vi "GuiderSetupGUI.vi"() -> ()   [LabVIEW 2018]
uses:
  GuiderSetup/GuiderSetup.lvclass
  C:/Users/devstaff/sparc4/s4gui/Versao ZeroMQ REQ-REP/SPARC4_GUI -20241104/S4GUI/S4GUI.lvclass
  S4GUI/S4GUI.lvclass/S4GUI.ctl
  Instrument/Instrument.lvclass/Instrument.ctl
  Device/Optics/Optics.lvclass/Optics.ctl
  Device/Optics/Opt_Continuous/Opt_Continuous.lvclass
  C:/Users/devstaff/sparc4/s4gui/Versao ZeroMQ REQ-REP/SPARC4_GUI -20241104/Device/Optics/Optics.lvclass
  Instrument/Instrument.lvclass
  AG/AG.lvclass
  Device/angles/angles.lvclass
  S4GUI/S4GUI.lvclass
  Device/Optics/Optics.lvclass
  StateMachine/State Machine.lvclass
panel:
  out "GUI version":string
  in  "Tab Focus":enum32{"FOCUS", "Config"}(tab)
  in  "Guider Focus Target":dbl caption="Target" min=0.0 max=24.9 step=0.1
  in  "GOTO GFOC":bool
  in  "STOP GFOC":bool
  in  "GFOC IN":bool
  in  "GFOC OUT":bool
  out "Pos GFOC":dbl caption="Position (mm)" format="%3_4g"
  out "GFOC status":bool
  in  "Guider Focus Incr":dbl caption="Increment" min=0.0 max=5.0 step=0.01 format="%#2_4g"
  in  "Set Focus by Mode":bool
  in  "Focus by Mode":T1={"Phot."=17.0, "Polarim"=7.0, "Efficiency"=0.0, "Instrumental"=0.0}
  out "AG connection":bool caption="AG"
  in  "Rotator":dbl caption="ROTATOR"
  out "loop max (ms)":u32
  out "loop time (ms)":u32
  in  "Guider Mirror Veloc":dbl=1.0 caption="Veloc. (1-30)" min=1.0 max=30.0 step=1.0
  out "GMIR status":bool
  out "ICS connection":bool caption="ICS"
  out "error out":errorcluster
  out "Pos GMIR":dbl caption="Position (deg)" format="%-3_4g"
  in  "RUN GMIR":bool
  in  "STOP GMIR":bool
  in  "GOTO GMIR":bool
  in  "Guider Mirror Target":dbl caption="Target"
  in  "stop":bool
  in  "GuiderSetup.lvclass":refnum<class "GuiderSetup.lvclass">
  # "GUIDER SETUP"
  # "MIRROR"
  # "deg"
  # "deg/s"
  # "FOCUS"
  # "mm"
  # "mm"
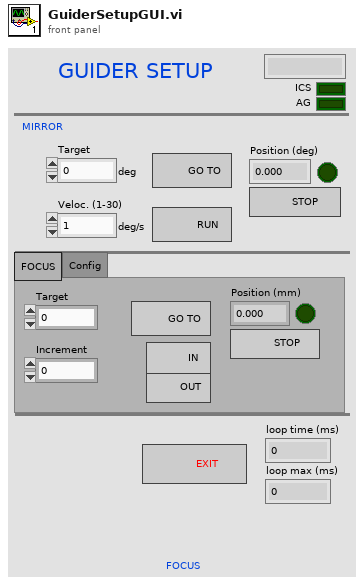
[diagram p1: front panel]
types:
  T1 = cluster{"Phot.":dbl, "Polarim":dbl, "Efficiency":dbl, "Instrumental":dbl}
  T2 = cluster{"Trigger Mode Status":string, "String output":string, "Instrument Status":cluster{"WPROT pos":dbl, "WPSEL pos":dbl, "GMIR pos":dbl, "GFOC pos":dbl, "CALW pos":dbl, "ASEL pos":dbl, "mode":bool, "String Status":string, "connection":bool, "operational":bool}, "Sync Box State":i32, "Trigger General Status":string, "Instrument States":cluster{"WPSEL State":i32, "WPROT State":i32, "CALW State":i32, "ASEL State":i32, "GMIR State":i32, "GFOC State":i32}, "Instrument Pos Names":cluster{"WPROT posname":string, "WPSEL posname":string, "CALW posname":string, "ASEL posname":string}, "ChannelA_Status":cluster{"Current exp":dbl, "Frames done":u32, "LastFileImage":string, "CamStatus":string, "Run state":u32, "connection":bool, "Cooler ON/OFF":i16, "Currently temperature":i16, "Temperature Status":string, "target  temp":i16, "conf runing":bool, "FT":bool, "UsedDisk":u16, "operational":bool}, "WPROT seq":u16, "ChannelB_Status":cluster{"Current exp":dbl, "Frames done":u32, "LastFileImage":string, "CamStatus":string, "Run state":u32, "connection":bool, "Cooler ON/OFF":i16, "Currently temperature":i16, "Temperature Status":string, "target  temp":i16, "conf runing":bool, "FT":bool, "UsedDisk":u16, "operational":bool}, "ChannelC_Status":cluster{"Current exp":dbl, "Frames done":u32, "LastFileImage":string, "CamStatus":string, "Run state":u32, "connection":bool, "Cooler ON/OFF":i16, "Currently temperature":i16, "Temperature Status":string, "target  temp":i16, "conf runing":bool, "FT":bool, "UsedDisk":u16, "operational":bool}, "ChannelD_Status":cluster{"Current exp":dbl, "Frames done":u32, "LastFileImage":string, "CamStatus":string, "Run state":u32, "connection":bool, "Cooler ON/OFF":i16, "Currently temperature":i16, "Temperature Status":string, "target  temp":i16, "conf runing":bool, "FT":bool, "UsedDisk":u16, "operational":bool}, "ChannelA_CCD":cluster{"ACQUISITION_MODE":u8, "TRIGGER_MODE":u8, "READ_MODE":u8, "PREAMP":u8, "READOUT_RATE":u8, "VERTICAL_SHIFT_SPEED":u8, "EM_MODE":u8, "EM_GAIN":u16, "SHUTTER_MODE":u8, "SHUTTER_TTL":u8, "SHUTTER_OPENNING_TIME":u16, "SHUTTER_CLOSING_TIME":u16, "VBIN":u16, "HBIN":u16, "INITIAL_LINE":u16, "INITIAL_COLUMN":u16, "FINAL_LINE":u16, "FINAL_COLUMN":u16, "FRAME_TRANSFER":bool, "VERTICAL_CLOCK_VOLTAGE":u8, "AD_CHANNEL":u32}, "ChannelB_CCD ":cluster{"ACQUISITION_MODE":u8, "TRIGGER_MODE":u8, "READ_MODE":u8, "PREAMP":u8, "READOUT_RATE":u8, "VERTICAL_SHIFT_SPEED":u8, "EM_MODE":u8, "EM_GAIN":u16, "SHUTTER_MODE":u8, "SHUTTER_TTL":u8, "SHUTTER_OPENNING_TIME":u16, "SHUTTER_CLOSING_TIME":u16, "VBIN":u16, "HBIN":u16, "INITIAL_LINE":u16, "INITIAL_COLUMN":u16, "FINAL_LINE":u16, "FINAL_COLUMN":u16, "FRAME_TRANSFER":bool, "VERTICAL_CLOCK_VOLTAGE":u8, "AD_CHANNEL":u32}, "ChannelC_CCD":cluster{"ACQUISITION_MODE":u8, "TRIGGER_MODE":u8, "READ_MODE":u8, "PREAMP":u8, "READOUT_RATE":u8, "VERTICAL_SHIFT_SPEED":u8, "EM_MODE":u8, "EM_GAIN":u16, "SHUTTER_MODE":u8, "SHUTTER_TTL":u8, "SHUTTER_OPENNING_TIME":u16, "SHUTTER_CLOSING_TIME":u16, "VBIN":u16, "HBIN":u16, "INITIAL_LINE":u16, "INITIAL_COLUMN":u16, "FINAL_LINE":u16, "FINAL_COLUMN":u16, "FRAME_TRANSFER":bool, "VERTICAL_CLOCK_VOLTAGE":u8, "AD_CHANNEL":u32}, "ChannelD_CCD":cluster{"ACQUISITION_MODE":u8, "TRIGGER_MODE":u8, "READ_MODE":u8, "PREAMP":u8, "READOUT_RATE":u8, "VERTICAL_SHIFT_SPEED":u8, "EM_MODE":u8, "EM_GAIN":u16, "SHUTTER_MODE":u8, "SHUTTER_TTL":u8, "SHUTTER_OPENNING_TIME":u16, "SHUTTER_CLOSING_TIME":u16, "VBIN":u16, "HBIN":u16, "INITIAL_LINE":u16, "INITIAL_COLUMN":u16, "FINAL_LINE":u16, "FINAL_COLUMN":u16, "FRAME_TRANSFER":bool, "VERTICAL_CLOCK_VOLTAGE":u8, "AD_CHANNEL":u32}, "CHA_Checked Params":cluster{"ACQUISITION_MODE":bool, "TRIGGER_MODE":bool, "READ_MODE":bool, "PREAMP":bool, "READOUT_RATE":bool, "VERTICAL_SHIFT_SPEED":bool, "EM_MODE":bool, "EM_GAIN":bool, "SHUTTER_MODE":bool, "SHUTTER_TTL":bool, "SHUTTER_OPENING_TIME":bool, "SHUTTER_CLOSING_TIME":bool, "VBIN":bool, "HBIN":bool, "INITIAL_LINE":bool, "INITIAL_COLUMN":bool, "FINAL_LINE":bool, "FINAL_COLUMN":bool, "FRAME_TRANSFER":bool, "VERTICAL_CLOCK_VOLTAGE":bool, "AD_CHANNEL":bool}, "CHB_Checked Params":cluster{"ACQUISITION_MODE":bool, "TRIGGER_MODE":bool, "READ_MODE":bool, "PREAMP":bool, "READOUT_RATE":bool, "VERTICAL_SHIFT_SPEED":bool, "EM_MODE":bool, "EM_GAIN":bool, "SHUTTER_MODE":bool, "SHUTTER_TTL":bool, "SHUTTER_OPENING_TIME":bool, "SHUTTER_CLOSING_TIME":bool, "VBIN":bool, "HBIN":bool, "INITIAL_LINE":bool, "INITIAL_COLUMN":bool, "FINAL_LINE":bool, "FINAL_COLUMN":bool, "FRAME_TRANSFER":bool, "VERTICAL_CLOCK_VOLTAGE":bool, "AD_CHANNEL":bool}, "CHC_Checked Params":cluster{"ACQUISITION_MODE":bool, "TRIGGER_MODE":bool, "READ_MODE":bool, "PREAMP":bool, "READOUT_RATE":bool, "VERTICAL_SHIFT_SPEED":bool, "EM_MODE":bool, "EM_GAIN":bool, "SHUTTER_MODE":bool, "SHUTTER_TTL":bool, "SHUTTER_OPENING_TIME":bool, "SHUTTER_CLOSING_TIME":bool, "VBIN":bool, "HBIN":bool, "INITIAL_LINE":bool, "INITIAL_COLUMN":bool, "FINAL_LINE":bool, "FINAL_COLUMN":bool, "FRAME_TRANSFER":bool, "VERTICAL_CLOCK_VOLTAGE":bool, "AD_CHANNEL":bool}, "CHD_Checked Params":cluster{"ACQUISITION_MODE":bool, "TRIGGER_MODE":bool, "READ_MODE":bool, "PREAMP":bool, "READOUT_RATE":bool, "VERTICAL_SHIFT_SPEED":bool, "EM_MODE":bool, "EM_GAIN":bool, "SHUTTER_MODE":bool, "SHUTTER_TTL":bool, "SHUTTER_OPENING_TIME":bool, "SHUTTER_CLOSING_TIME":bool, "VBIN":bool, "HBIN":bool, "INITIAL_LINE":bool, "INITIAL_COLUMN":bool, "FINAL_LINE":bool, "FINAL_COLUMN":bool, "FRAME_TRANSFER":bool, "VERTICAL_CLOCK_VOLTAGE":bool, "AD_CHANNEL":bool}, "Trigger_connection":bool, "TCSPD_connection":bool, "TCS extended":string, "TCS id":u32, "S4ICS id":u32, "focus pos":i32, "Focus_connection":bool, "WS_connection":bool, "weather status":cluster{"broker":string, "version":string, "date":string, "hour":string, "outHumidity":string, "inHumidity":string, "inTemp":string, "outTemp":string, "windSpeed":string, "windDirection":string, "pressure":string, "dewOut":string, "dewIn":string, "leaf":string, "rain":string, "windChill":string}, "GS STATUS cluster":cluster{"FocusPhot":dbl, "FocusPolar":dbl, "FocusEffic":dbl, "FocusInstrum":dbl, "ICS":bool, "AG":bool, "BROKER":string}, "TCSPD_operational":bool, "Focus_operational":bool}
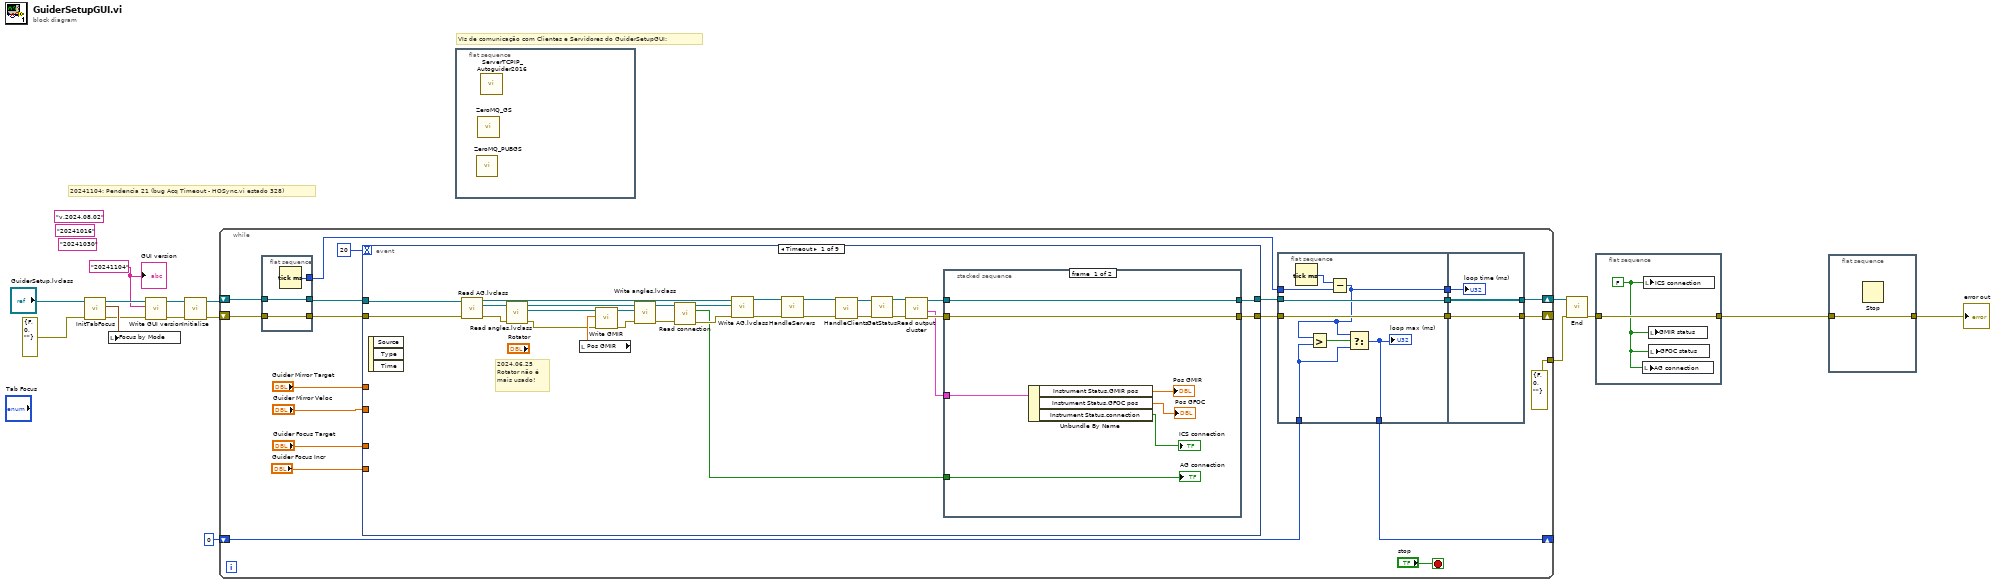
[diagram p0: block diagram]
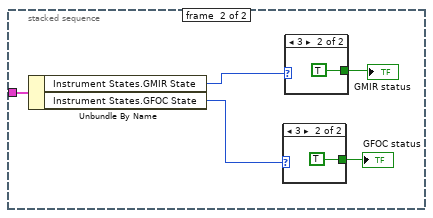
[diagram p2: hidden frame]
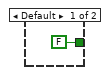
[diagram p3: hidden frame]
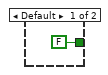
[diagram p4: hidden frame]
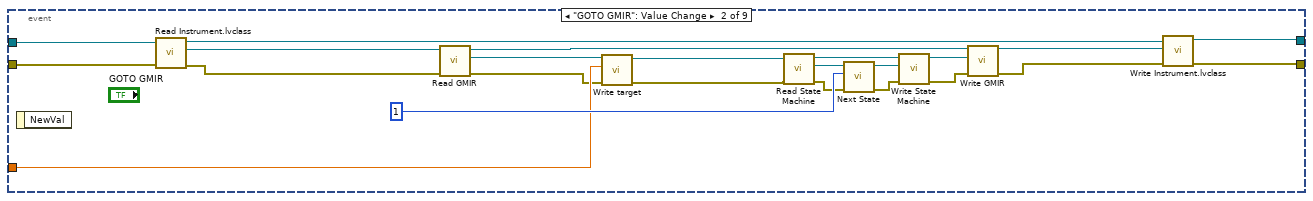
[diagram p5: hidden frame]
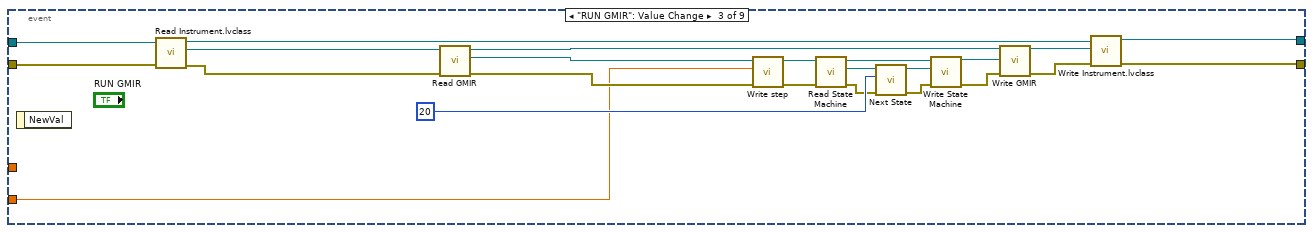
[diagram p6: hidden frame]
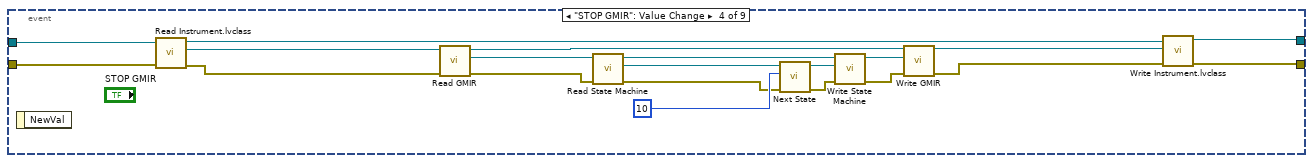
[diagram p7: hidden frame]
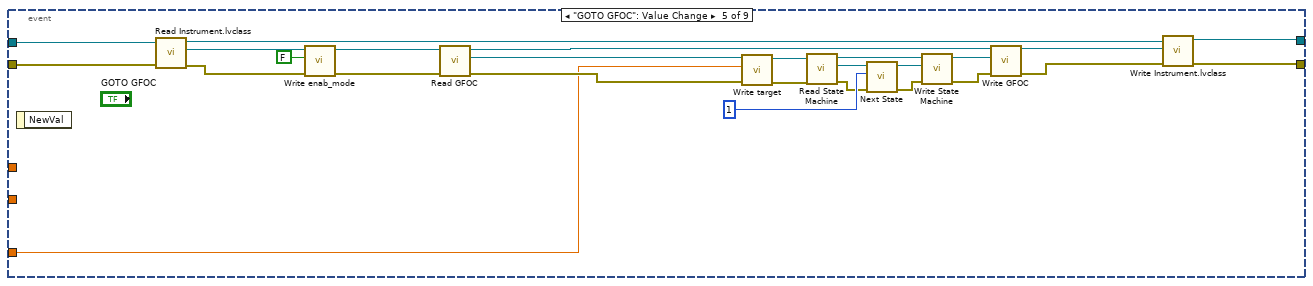
[diagram p8: hidden frame]
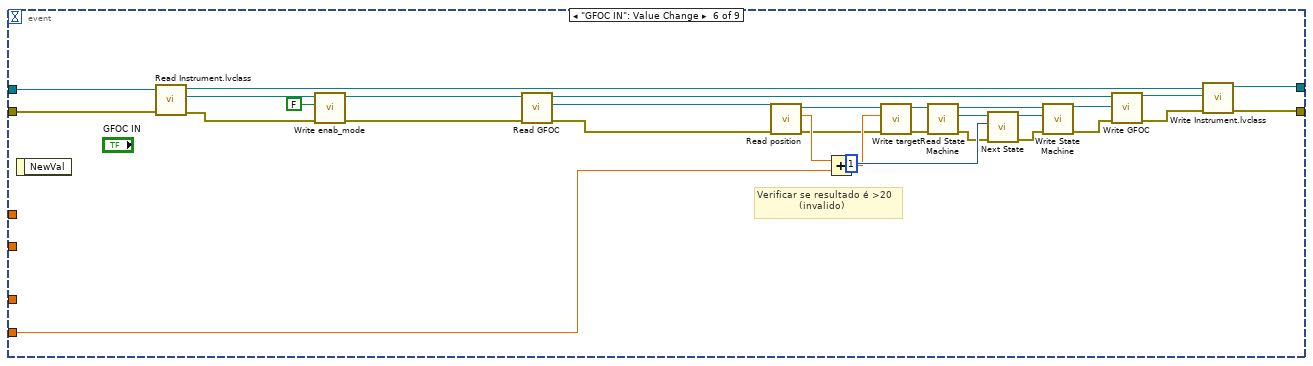
[diagram p9: hidden frame]
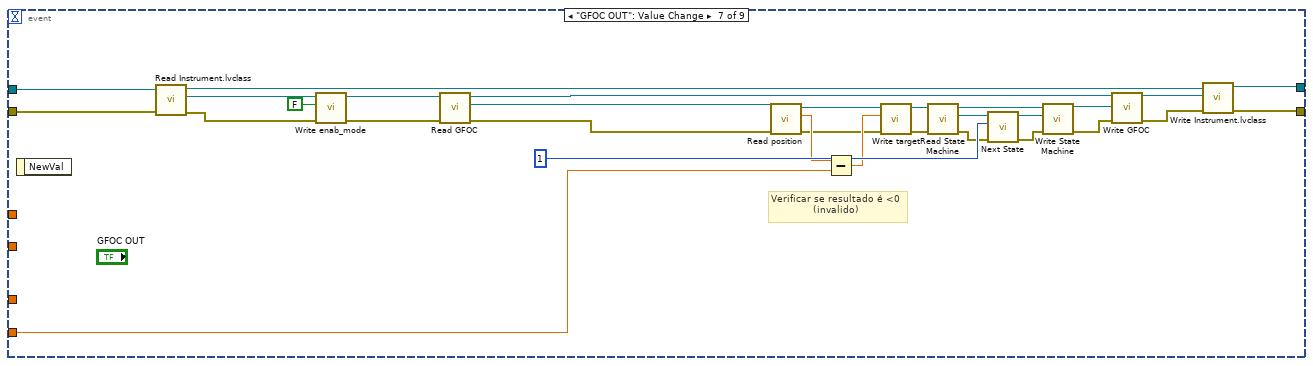
[diagram p10: hidden frame]
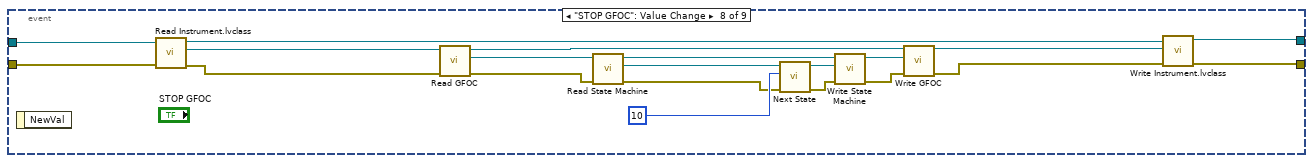
[diagram p11: hidden frame]
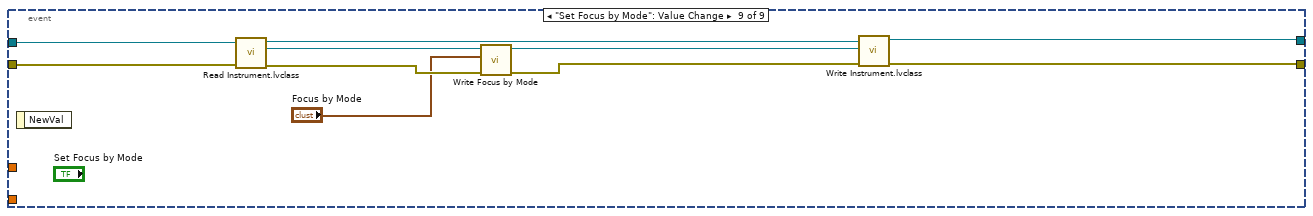
[diagram p12: hidden frame]
diagram:
  (unwired) "20241030" ("GUI version")
  (unwired) "20241016" ("GUI version")
  w1 = "20241104" ("GUI version")
  (unwired) "v.2024.08.02" ("GUI version")
  # "20241104: Pendencia 21 (bug Acq Timeout - HOSync.vi estado 328)"
  # "VIs de comunicação com Clientes e Servidores do GuiderSetupGUI:"
  n1 = call-dynamic "InitTabFocus.vi"("error in (no error)"=errorcluster {"status"=FALSE, "code"=0, "source"=""}, "GuiderSetup in"="GuiderSetup.lvclass") -> ("error out"=w5:errorcluster, "output cluster"=w8:T1, "GuiderSetup out"=w7:refnum<class "GuiderSetup.lvclass">)  [unwired: 7 in]
  n2 = local write "Focus by Mode"(w8) -> ()
  n3 = call-dynamic "Write GUI version.vi"("error in (no error)"=w5, "GUI version"=w1, "S4GUI in"=w7) -> ("error out"=w4:errorcluster, "S4GUI out"=w6:refnum<class "GuiderSetup.lvclass">)  [unwired: 7 in]
  n4 = call-dynamic "Initialize.vi"("error in (no error)"=w4, "S4ACS_GUI in"=w6) -> ("error out"=w15:errorcluster, "S4ACS_GUI out"=w16:refnum<class "GuiderSetup.lvclass">)  [unwired: 8 in]
  n5 = while {
    shift-right: [w24] -> w14
    shift-left: w16 -> [w31]
    shift-right: [w25] -> _
    shift-left: w15 -> [w30]
    shift-right: [w19] -> _
    shift-left: u32 0 -> [w18]
    tunnel: [errorcluster {"status"=FALSE, "code"=0, "source"=""} ("error in (no error)")] -> w11
    stop <- "stop" stop-if-true
    n6 = flat-sequence {
      tunnel: [w51] -> w20
      tunnel: w31 -> [w50]
      tunnel: w30 -> [w49]
      tunnel: [w50] -> w29
      tunnel: [w49] -> w28
      frame #0 {
        n7 = Tick Count (ms)() -> (millisecond timer value=w51:u32)
      }
    }
    n8 = event shown="[0] Timeout" {
      selector: _ -> [_ _ _ _ _ _ _ _ _]
      dyn-events: _ -> [_ _ _ _ _ _ _ _ _]
      timeout: 20 -> [_ _ _ _ _ _ _ _ _]
      tunnel: w29 -> [w80 w119 w142 w162 w188 w218 w248 w268 w278]
      tunnel: [w64 w117 w140 w160 w186 w216 w246 w266 w276] -> w27
      tunnel: w28 -> [w79 w113 w136 w156 w183 w213 w243 w262 w275]
      tunnel: [w61 w110 w133 w153 w181 w211 w241 w259 w274] -> w26
      tunnel: "Guider Mirror Veloc" -> [_ _ w120 _ _ _ _ _ _]
      tunnel: "Guider Mirror Target" -> [_ w99 _ _ _ _ _ _ _]
      tunnel: "Guider Focus Target" -> [_ _ _ _ w168 _ _ _ _]
      tunnel: "Guider Focus Incr" -> [_ _ _ _ _ w194 w224 _ _]
      event Timeout {
        # "2024.06.25\nRotator não é \nmais usado!"
        n9 = event-data() -> ()  [unwired: 1 in, 3 out]
        n10 = call-dynamic "Read AG.lvclass.vi"("error in (no error)"=w79, "GuiderSetup in"=w80) -> ("error out"=w74:errorcluster, "AG.lvclass"=w77:refnum<class "AG.lvclass">, "GuiderSetup out"=w78:refnum<class "GuiderSetup.lvclass">)  [unwired: 7 in]
        n11 = call-dynamic "Read angles.lvclass.vi"("error in (no error)"=w74, "AG in"=w77) -> ("error out"=w62:errorcluster, "angles.lvclass"=w63:refnum<class "angles.lvclass">, "AG out"=w76:refnum<class "AG.lvclass">)  [unwired: 7 in]
        n12 = local read "Pos GMIR"() -> (w72:dbl)
        n13 = call-dynamic "Write GMIR.vi"("error in (no error)"=w62, "GMIR"=w72, "angles in"=w63) -> ("error out"=w73:errorcluster, "angles out"=w75:refnum<class "angles.lvclass">)  [unwired: 7 in]
        n14 = call-dynamic "Write angles.lvclass.vi"("error in (no error)"=w73, "angles.lvclass"=w75, "AG in"=w76) -> ("error out"=w67:errorcluster, "AG out"=w69:refnum<class "AG.lvclass">)  [unwired: 7 in]
        n15 = call-dynamic "Read connection.vi"("error in (no error)"=w67, "Client in"=w69) -> ("error out"=w66:errorcluster, "connection"=w65:bool, "Client out"=w68:refnum<class "AG.lvclass">)  [unwired: 7 in]
        n16 = call-dynamic "Write AG.lvclass.vi"("error in (no error)"=w66, "AG.lvclass"=w68, "GuiderSetup in"=w78) -> ("error out"=w71:errorcluster, "GuiderSetup out"=w70:refnum<class "GuiderSetup.lvclass">)  [unwired: 7 in]
        n17 = call-dynamic "HandleServers.vi"("error in (no error)"=w71, "S4ACS_GUI in"=w70) -> ("error out"=w58:errorcluster, "S4ACS_GUI out"=w60:refnum<class "GuiderSetup.lvclass">)  [unwired: 8 in]
        n18 = call-dynamic "HandleClients.vi"("error in (no error)"=w58, "GuiderSetup in"=w60) -> ("error out"=w57:errorcluster, "GuiderSetup out"=w59:refnum<class "GuiderSetup.lvclass">)  [unwired: 8 in]
        n19 = call-dynamic "GetStatus.vi"("error in (no error)"=w57, "GS in"=w59) -> ("error out"=w54:errorcluster, "GS out"=w56:refnum<class "GuiderSetup.lvclass">)  [unwired: 8 in]
        n20 = call-dynamic "Read output cluster.vi"("error in (no error)"=w54, "S4GUI in"=w56) -> ("error out"=w53:errorcluster, "output cluster"=w52:T2, "S4GUI out"=w55:refnum<class "GuiderSetup.lvclass">)  [unwired: 7 in]
        n21 = stacked-sequence {
          tunnel: w65 -> [w84 _]
          tunnel: w55 -> [w83 _]
          tunnel: w53 -> [w82 _]
          tunnel: [w83 _] -> w64
          tunnel: [w82 _] -> w61
          tunnel: w52 -> [w81 w88]
          frame #0 {
            n22 = Unbundle By Name(w81) -> ("Instrument Status.GMIR pos"=→"Pos GMIR":dbl, "Instrument Status.GFOC pos"=→"Pos GFOC":dbl, "Instrument Status.connection"=→"ICS connection":bool)
            "AG connection" <- w84
          }
          frame #1 {
            n23 = Unbundle By Name(w88) -> ("Instrument States.GMIR State"=w92:i32, "Instrument States.GFOC State"=w90:i32)
            n24 = case shown="3" w90 {
              tunnel: [FALSE TRUE] -> w89
              frame Default {
              }
              frame 3 {
              }
            }
            "GFOC status" <- w89
            n25 = case shown="3" w92 {
              tunnel: [FALSE TRUE] -> w91
              frame Default {
              }
              frame 3 {
              }
            }
            "GMIR status" <- w91
          }
        }
      }
      event "GOTO GMIR": Value Change {
        n26 = event-data() -> ()  [unwired: 1 in, 1 out]
        n27 = call "Read Instrument.lvclass.vi"("error in (no error)"=w113, "S4ACS_GUI in"=w119) -> ("error out"=w112:errorcluster, "Instrument.lvclass"=w116:refnum<class "Instrument.lvclass">, "S4ACS_GUI out"=w118:refnum<class "GuiderSetup.lvclass">)  [unwired: 7 in]
        n28 = call "Read GMIR.vi"("error in (no error)"=w112, "Instrument in"=w116) -> ("error out"=w98:errorcluster, "Opt_Continuous.lvclass"=w101:refnum<class "Opt_Continuous.lvclass">, "Instrument out"=w115:refnum<class "Instrument.lvclass">)  [unwired: 7 in]
        n29 = call "Write target.vi"("error in (no error)"=w98, "target"=w99, "Optics in"=w101) -> ("error out"=w97:errorcluster, "Optics out"=w100:refnum<class "Opt_Continuous.lvclass">)  [unwired: 7 in]
        n30 = call-dynamic "Read State Machine.vi"("error in (no error)"=w97, "Device in"=w100) -> ("error out"=w104:errorcluster, "State Machine.lvclass"=w107:refnum<class "State Machine.lvclass">, "Device out"=w109:refnum<class "Opt_Continuous.lvclass">)  [unwired: 7 in]
        n31 = call "Next State.vi"("error in (no error)"=w104, "New_State"=1, "State Machine in"=w107) -> ("error out"=w103:errorcluster, "State Machine out"=w106:refnum<class "State Machine.lvclass">)  [unwired: 7 in]
        n32 = call-dynamic "Write State Machine.vi"("error in (no error)"=w103, "State Machine.lvclass"=w106, "Device in"=w109) -> ("error out"=w102:errorcluster, "Device out"=w108:refnum<class "Opt_Continuous.lvclass">)  [unwired: 7 in]
        n33 = call "Write GMIR.vi"("error in (no error)"=w102, "Opt_Continuous.lvclass"=w108, "Instrument in"=w115) -> ("error out"=w111:errorcluster, "Instrument out"=w114:refnum<class "Instrument.lvclass">)  [unwired: 7 in]
        n34 = call "Write Instrument.lvclass.vi"("error in (no error)"=w111, "Instrument.lvclass"=w114, "S4ACS_GUI in"=w118) -> ("error out"=w110:errorcluster, "S4ACS_GUI out"=w117:refnum<class "GuiderSetup.lvclass">)  [unwired: 7 in]
      }
      event "RUN GMIR": Value Change {
        n35 = event-data() -> ()  [unwired: 1 in, 1 out]
        n36 = call "Read Instrument.lvclass.vi"("error in (no error)"=w136, "S4ACS_GUI in"=w142) -> ("error out"=w135:errorcluster, "Instrument.lvclass"=w139:refnum<class "Instrument.lvclass">, "S4ACS_GUI out"=w141:refnum<class "GuiderSetup.lvclass">)  [unwired: 7 in]
        n37 = call "Read GMIR.vi"("error in (no error)"=w135, "Instrument in"=w139) -> ("error out"=w123:errorcluster, "Opt_Continuous.lvclass"=w124:refnum<class "Opt_Continuous.lvclass">, "Instrument out"=w138:refnum<class "Instrument.lvclass">)  [unwired: 7 in]
        n38 = call-dynamic "Write step.vi"("error in (no error)"=w123, "step"=w120, "Optics in"=w124) -> ("error out"=w122:errorcluster, "Optics out"=w121:refnum<class "Opt_Continuous.lvclass">)  [unwired: 7 in]
        n39 = call-dynamic "Read State Machine.vi"("error in (no error)"=w122, "Device in"=w121) -> ("error out"=w127:errorcluster, "State Machine.lvclass"=w130:refnum<class "State Machine.lvclass">, "Device out"=w132:refnum<class "Opt_Continuous.lvclass">)  [unwired: 7 in]
        n40 = call "Next State.vi"("error in (no error)"=w127, "New_State"=20, "State Machine in"=w130) -> ("error out"=w126:errorcluster, "State Machine out"=w129:refnum<class "State Machine.lvclass">)  [unwired: 7 in]
        n41 = call-dynamic "Write State Machine.vi"("error in (no error)"=w126, "State Machine.lvclass"=w129, "Device in"=w132) -> ("error out"=w125:errorcluster, "Device out"=w131:refnum<class "Opt_Continuous.lvclass">)  [unwired: 7 in]
        n42 = call "Write GMIR.vi"("error in (no error)"=w125, "Opt_Continuous.lvclass"=w131, "Instrument in"=w138) -> ("error out"=w134:errorcluster, "Instrument out"=w137:refnum<class "Instrument.lvclass">)  [unwired: 7 in]
        n43 = call "Write Instrument.lvclass.vi"("error in (no error)"=w134, "Instrument.lvclass"=w137, "S4ACS_GUI in"=w141) -> ("error out"=w133:errorcluster, "S4ACS_GUI out"=w140:refnum<class "GuiderSetup.lvclass">)  [unwired: 7 in]
      }
      event "STOP GMIR": Value Change {
        n44 = event-data() -> ()  [unwired: 1 in, 1 out]
        n45 = call "Read Instrument.lvclass.vi"("error in (no error)"=w156, "S4ACS_GUI in"=w162) -> ("error out"=w155:errorcluster, "Instrument.lvclass"=w159:refnum<class "Instrument.lvclass">, "S4ACS_GUI out"=w161:refnum<class "GuiderSetup.lvclass">)  [unwired: 7 in]
        n46 = call "Read GMIR.vi"("error in (no error)"=w155, "Instrument in"=w159) -> ("error out"=w146:errorcluster, "Opt_Continuous.lvclass"=w152:refnum<class "Opt_Continuous.lvclass">, "Instrument out"=w158:refnum<class "Instrument.lvclass">)  [unwired: 7 in]
        n47 = call-dynamic "Read State Machine.vi"("error in (no error)"=w146, "Device in"=w152) -> ("error out"=w145:errorcluster, "State Machine.lvclass"=w149:refnum<class "State Machine.lvclass">, "Device out"=w151:refnum<class "Opt_Continuous.lvclass">)  [unwired: 7 in]
        n48 = call "Next State.vi"("error in (no error)"=w145, "New_State"=10, "State Machine in"=w149) -> ("error out"=w144:errorcluster, "State Machine out"=w148:refnum<class "State Machine.lvclass">)  [unwired: 7 in]
        n49 = call-dynamic "Write State Machine.vi"("error in (no error)"=w144, "State Machine.lvclass"=w148, "Device in"=w151) -> ("error out"=w143:errorcluster, "Device out"=w150:refnum<class "Opt_Continuous.lvclass">)  [unwired: 7 in]
        n50 = call "Write GMIR.vi"("error in (no error)"=w143, "Opt_Continuous.lvclass"=w150, "Instrument in"=w158) -> ("error out"=w154:errorcluster, "Instrument out"=w157:refnum<class "Instrument.lvclass">)  [unwired: 7 in]
        n51 = call "Write Instrument.lvclass.vi"("error in (no error)"=w154, "Instrument.lvclass"=w157, "S4ACS_GUI in"=w161) -> ("error out"=w153:errorcluster, "S4ACS_GUI out"=w160:refnum<class "GuiderSetup.lvclass">)  [unwired: 7 in]
      }
      event "GOTO GFOC": Value Change {
        n52 = event-data() -> ()  [unwired: 1 in, 1 out]
        n53 = call "Read Instrument.lvclass.vi"("error in (no error)"=w183, "S4ACS_GUI in"=w188) -> ("error out"=w166:errorcluster, "Instrument.lvclass"=w167:refnum<class "Instrument.lvclass">, "S4ACS_GUI out"=w187:refnum<class "GuiderSetup.lvclass">)  [unwired: 7 in]
        n54 = call-dynamic "Write enab_mode.vi"("error in (no error)"=w166, "enab_mode"=FALSE, "Instrument in"=w167) -> ("error out"=w163:errorcluster, "Instrument out"=w164:refnum<class "Instrument.lvclass">)  [unwired: 7 in]
        n55 = call "Read GFOC.vi"("error in (no error)"=w163, "Instrument in"=w164) -> ("error out"=w170:errorcluster, "Opt_Continuous.lvclass"=w172:refnum<class "Opt_Continuous.lvclass">, "Instrument out"=w185:refnum<class "Instrument.lvclass">)  [unwired: 7 in]
        n56 = call "Write target.vi"("error in (no error)"=w170, "target"=w168, "Optics in"=w172) -> ("error out"=w169:errorcluster, "Optics out"=w171:refnum<class "Opt_Continuous.lvclass">)  [unwired: 7 in]
        n57 = call-dynamic "Read State Machine.vi"("error in (no error)"=w169, "Device in"=w171) -> ("error out"=w175:errorcluster, "State Machine.lvclass"=w178:refnum<class "State Machine.lvclass">, "Device out"=w180:refnum<class "Opt_Continuous.lvclass">)  [unwired: 7 in]
        n58 = call "Next State.vi"("error in (no error)"=w175, "New_State"=1, "State Machine in"=w178) -> ("error out"=w174:errorcluster, "State Machine out"=w177:refnum<class "State Machine.lvclass">)  [unwired: 7 in]
        n59 = call-dynamic "Write State Machine.vi"("error in (no error)"=w174, "State Machine.lvclass"=w177, "Device in"=w180) -> ("error out"=w173:errorcluster, "Device out"=w179:refnum<class "Opt_Continuous.lvclass">)  [unwired: 7 in]
        n60 = call "Write GFOC.vi"("error in (no error)"=w173, "Opt_Continuous.lvclass"=w179, "Instrument in"=w185) -> ("error out"=w182:errorcluster, "Instrument out"=w184:refnum<class "Instrument.lvclass">)  [unwired: 7 in]
        n61 = call "Write Instrument.lvclass.vi"("error in (no error)"=w182, "Instrument.lvclass"=w184, "S4ACS_GUI in"=w187) -> ("error out"=w181:errorcluster, "S4ACS_GUI out"=w186:refnum<class "GuiderSetup.lvclass">)  [unwired: 7 in]
      }
      event "GFOC IN": Value Change {
        # "Verificar se resultado é >20 \n              (invalido)"
        n62 = event-data() -> ()  [unwired: 1 in, 1 out]
        n63 = call "Read Instrument.lvclass.vi"("error in (no error)"=w213, "S4ACS_GUI in"=w218) -> ("error out"=w191:errorcluster, "Instrument.lvclass"=w192:refnum<class "Instrument.lvclass">, "S4ACS_GUI out"=w217:refnum<class "GuiderSetup.lvclass">)  [unwired: 7 in]
        n64 = call-dynamic "Write enab_mode.vi"("error in (no error)"=w191, "enab_mode"=FALSE, "Instrument in"=w192) -> ("error out"=w189:errorcluster, "Instrument out"=w190:refnum<class "Instrument.lvclass">)  [unwired: 7 in]
        n65 = call "Read GFOC.vi"("error in (no error)"=w189, "Instrument in"=w190) -> ("error out"=w195:errorcluster, "Opt_Continuous.lvclass"=w196:refnum<class "Opt_Continuous.lvclass">, "Instrument out"=w215:refnum<class "Instrument.lvclass">)  [unwired: 7 in]
        n66 = call "Read position.vi"("error in (no error)"=w195, "Optics in"=w196) -> ("error out"=w199:errorcluster, "position"=w202:dbl, "Optics out"=w200:refnum<class "Opt_Continuous.lvclass">)  [unwired: 7 in]
        n67 = Add(x=w202, y=w194) -> (x+y=w201:dbl)
        n68 = call "Write target.vi"("error in (no error)"=w199, "target"=w201, "Optics in"=w200) -> ("error out"=w198:errorcluster, "Optics out"=w197:refnum<class "Opt_Continuous.lvclass">)  [unwired: 7 in]
        n69 = call-dynamic "Read State Machine.vi"("error in (no error)"=w198, "Device in"=w197) -> ("error out"=w205:errorcluster, "State Machine.lvclass"=w208:refnum<class "State Machine.lvclass">, "Device out"=w210:refnum<class "Opt_Continuous.lvclass">)  [unwired: 7 in]
        n70 = call "Next State.vi"("error in (no error)"=w205, "New_State"=1, "State Machine in"=w208) -> ("error out"=w204:errorcluster, "State Machine out"=w207:refnum<class "State Machine.lvclass">)  [unwired: 7 in]
        n71 = call-dynamic "Write State Machine.vi"("error in (no error)"=w204, "State Machine.lvclass"=w207, "Device in"=w210) -> ("error out"=w203:errorcluster, "Device out"=w209:refnum<class "Opt_Continuous.lvclass">)  [unwired: 7 in]
        n72 = call "Write GFOC.vi"("error in (no error)"=w203, "Opt_Continuous.lvclass"=w209, "Instrument in"=w215) -> ("error out"=w212:errorcluster, "Instrument out"=w214:refnum<class "Instrument.lvclass">)  [unwired: 7 in]
        n73 = call "Write Instrument.lvclass.vi"("error in (no error)"=w212, "Instrument.lvclass"=w214, "S4ACS_GUI in"=w217) -> ("error out"=w211:errorcluster, "S4ACS_GUI out"=w216:refnum<class "GuiderSetup.lvclass">)  [unwired: 7 in]
      }
      event "GFOC OUT": Value Change {
        # "Verificar se resultado é <0\n              (invalido)"
        n74 = event-data() -> ()  [unwired: 1 in, 1 out]
        n75 = call "Read Instrument.lvclass.vi"("error in (no error)"=w243, "S4ACS_GUI in"=w248) -> ("error out"=w221:errorcluster, "Instrument.lvclass"=w222:refnum<class "Instrument.lvclass">, "S4ACS_GUI out"=w247:refnum<class "GuiderSetup.lvclass">)  [unwired: 7 in]
        n76 = call-dynamic "Write enab_mode.vi"("error in (no error)"=w221, "enab_mode"=FALSE, "Instrument in"=w222) -> ("error out"=w219:errorcluster, "Instrument out"=w220:refnum<class "Instrument.lvclass">)  [unwired: 7 in]
        n77 = call "Read GFOC.vi"("error in (no error)"=w219, "Instrument in"=w220) -> ("error out"=w225:errorcluster, "Opt_Continuous.lvclass"=w226:refnum<class "Opt_Continuous.lvclass">, "Instrument out"=w245:refnum<class "Instrument.lvclass">)  [unwired: 7 in]
        n78 = call "Read position.vi"("error in (no error)"=w225, "Optics in"=w226) -> ("error out"=w229:errorcluster, "position"=w232:dbl, "Optics out"=w230:refnum<class "Opt_Continuous.lvclass">)  [unwired: 7 in]
        n79 = Subtract(x=w232, y=w224) -> (x-y=w231:dbl)
        n80 = call "Write target.vi"("error in (no error)"=w229, "target"=w231, "Optics in"=w230) -> ("error out"=w228:errorcluster, "Optics out"=w227:refnum<class "Opt_Continuous.lvclass">)  [unwired: 7 in]
        n81 = call-dynamic "Read State Machine.vi"("error in (no error)"=w228, "Device in"=w227) -> ("error out"=w235:errorcluster, "State Machine.lvclass"=w238:refnum<class "State Machine.lvclass">, "Device out"=w240:refnum<class "Opt_Continuous.lvclass">)  [unwired: 7 in]
        n82 = call "Next State.vi"("error in (no error)"=w235, "New_State"=1, "State Machine in"=w238) -> ("error out"=w234:errorcluster, "State Machine out"=w237:refnum<class "State Machine.lvclass">)  [unwired: 7 in]
        n83 = call-dynamic "Write State Machine.vi"("error in (no error)"=w234, "State Machine.lvclass"=w237, "Device in"=w240) -> ("error out"=w233:errorcluster, "Device out"=w239:refnum<class "Opt_Continuous.lvclass">)  [unwired: 7 in]
        n84 = call "Write GFOC.vi"("error in (no error)"=w233, "Opt_Continuous.lvclass"=w239, "Instrument in"=w245) -> ("error out"=w242:errorcluster, "Instrument out"=w244:refnum<class "Instrument.lvclass">)  [unwired: 7 in]
        n85 = call "Write Instrument.lvclass.vi"("error in (no error)"=w242, "Instrument.lvclass"=w244, "S4ACS_GUI in"=w247) -> ("error out"=w241:errorcluster, "S4ACS_GUI out"=w246:refnum<class "GuiderSetup.lvclass">)  [unwired: 7 in]
      }
      event "STOP GFOC": Value Change {
        n86 = event-data() -> ()  [unwired: 1 in, 1 out]
        n87 = call "Read Instrument.lvclass.vi"("error in (no error)"=w262, "S4ACS_GUI in"=w268) -> ("error out"=w261:errorcluster, "Instrument.lvclass"=w265:refnum<class "Instrument.lvclass">, "S4ACS_GUI out"=w267:refnum<class "GuiderSetup.lvclass">)  [unwired: 7 in]
        n88 = call "Read GFOC.vi"("error in (no error)"=w261, "Instrument in"=w265) -> ("error out"=w252:errorcluster, "Opt_Continuous.lvclass"=w258:refnum<class "Opt_Continuous.lvclass">, "Instrument out"=w264:refnum<class "Instrument.lvclass">)  [unwired: 7 in]
        n89 = call-dynamic "Read State Machine.vi"("error in (no error)"=w252, "Device in"=w258) -> ("error out"=w251:errorcluster, "State Machine.lvclass"=w255:refnum<class "State Machine.lvclass">, "Device out"=w257:refnum<class "Opt_Continuous.lvclass">)  [unwired: 7 in]
        n90 = call "Next State.vi"("error in (no error)"=w251, "New_State"=10, "State Machine in"=w255) -> ("error out"=w250:errorcluster, "State Machine out"=w254:refnum<class "State Machine.lvclass">)  [unwired: 7 in]
        n91 = call-dynamic "Write State Machine.vi"("error in (no error)"=w250, "State Machine.lvclass"=w254, "Device in"=w257) -> ("error out"=w249:errorcluster, "Device out"=w256:refnum<class "Opt_Continuous.lvclass">)  [unwired: 7 in]
        n92 = call "Write GFOC.vi"("error in (no error)"=w249, "Opt_Continuous.lvclass"=w256, "Instrument in"=w264) -> ("error out"=w260:errorcluster, "Instrument out"=w263:refnum<class "Instrument.lvclass">)  [unwired: 7 in]
        n93 = call "Write Instrument.lvclass.vi"("error in (no error)"=w260, "Instrument.lvclass"=w263, "S4ACS_GUI in"=w267) -> ("error out"=w259:errorcluster, "S4ACS_GUI out"=w266:refnum<class "GuiderSetup.lvclass">)  [unwired: 7 in]
      }
      event "Set Focus by Mode": Value Change {
        n94 = event-data() -> ()  [unwired: 1 in, 1 out]
        n95 = call "Read Instrument.lvclass.vi"("error in (no error)"=w275, "S4ACS_GUI in"=w278) -> ("error out"=w272:errorcluster, "Instrument.lvclass"=w273:refnum<class "Instrument.lvclass">, "S4ACS_GUI out"=w277:refnum<class "GuiderSetup.lvclass">)  [unwired: 7 in]
        n96 = call-dynamic "Write Focus by Mode.vi"("error in (no error)"=w272, "Focus by Mode"="Focus by Mode", "Instrument in"=w273) -> ("error out"=w270:errorcluster, "Instrument out"=w271:refnum<class "Instrument.lvclass">)  [unwired: 7 in]
        n97 = call "Write Instrument.lvclass.vi"("error in (no error)"=w270, "Instrument.lvclass"=w271, "S4ACS_GUI in"=w277) -> ("error out"=w274:errorcluster, "S4ACS_GUI out"=w276:refnum<class "GuiderSetup.lvclass">)  [unwired: 7 in]
      }
    }
    n98 = flat-sequence {
      tunnel: w27 -> [w45]
      tunnel: w26 -> [w44]
      tunnel: w20 -> [w43]
      tunnel: [w45] -> w23
      tunnel: [w44] -> w22
      tunnel: [w40] -> w21
      tunnel: [w39] -> w19
      tunnel: w18 -> [w38]
      tunnel: [w47] -> w25
      tunnel: [w48] -> w24
      tunnel: w23 -> [w48]
      tunnel: w22 -> [w47]
      tunnel: w21 -> [w46]
      frame #0 {
        n99 = Tick Count (ms)() -> (millisecond timer value=w42:u32)
        n100 = Subtract(x=w42, y=w43) -> (x-y=w40:u32)
        n101 = Greater?(x=w40, y=w38) -> (0:w41:bool)
        n102 = Select(t=w40, s=w41, f=w38) -> (s? t:f=w39:u32)
        "loop max (ms)" <- w39
      }
      frame #1 {
        "loop time (ms)" <- w46
      }
    }
  }
  n103 = flat-sequence {
    frame #0 {
      n104 = call "ZeroMQ_PUBGS.vi"() -> ()  [unwired: 12 in]
      n105 = call "ZeroMQ_GS.vi"() -> ()  [unwired: 12 in]
      n106 = call "ServerTCPIP_Autoguider2016.vi"() -> ()  [unwired: 12 in]
    }
  }
  n107 = call-dynamic "End.vi"("error in (no error)"=w11, "S4ACS_GUI in"=w14) -> ("error out"=w12:errorcluster)  [unwired: 8 in, 1 out]
  n108 = flat-sequence {
    tunnel: w12 -> [w280]
    tunnel: [w280] -> w3
    frame #0 {
      w279 = FALSE ("ICS connection")
      n109 = local write "AG connection"(w279) -> ()
      n110 = local write "ICS connection"(w279) -> ()
      n111 = local write "GMIR status"(w279) -> ()
      n112 = local write "GFOC status"(w279) -> ()
    }
  }
  n113 = flat-sequence {
    tunnel: w3 -> [w281]
    tunnel: [w281] -> w2
    frame #0 {
      n114 = Stop() -> ()  [unwired: 1 in]
    }
  }
  "error out" <- w2
  "GUI version" <- w1
